vi "oa_If Param Changed, Set Reset True (1 Channel).vi"(0 "scaled signal in [EU]":waveform(dbl)={"t0"=timestamp(0 s since 1904-01-01), "dt"=0.0, "Y"=[]}, 1 "reset in":bool=TRUE, 5 "speed profile":T1 {"speed [RPM]" format="%.2f"; "time [s]" format="%.2f"}, 7 "pulse/revolution in (1)":i32=1, 9 "max order in (auto)":dbl, 11 "error in (no error)":errorcluster, 12 "analysis method in":u16(ring) items=["fast", "accurate"]) -> (3 "reset out":bool=TRUE, 4 "scaled signal out [EU]":waveform(dbl), 6 "speed profile out":T1 {"speed [RPM]" format="%.2f"; "time [s]" format="%.2f"}, 8 "pulse/revolution out (1)":i32=1, 10 "max order out (auto)":dbl, 14 "analysis method out":u16(ring) items=["fast", "accurate"], 15 "error out":errorcluster)   [LabVIEW 2017, in "SoundVib_Resampling.lvlib"]
uses:
  <vilib>/addons/Sound and Vibration/Order Analysis/Resample Order Tracking/SoundVib_Resampling.lvlib
  <vilib>/addons/Sound and Vibration/Order Analysis/Tach Process/SubVIs/speed profile.ctl
  <vilib>/addons/Sound and Vibration/Order Analysis/Tach Process/SoundVib_TachProcess.lvlib
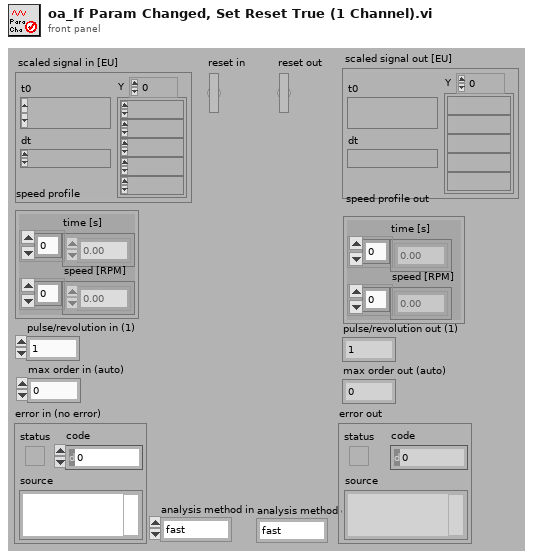
[diagram p1: front panel]
types:
  T1 = typedef "SoundVib_TachProcess.lvlib/speed profile.ctl" = cluster{"time [s]":dbl[], "speed [RPM]":dbl[]}
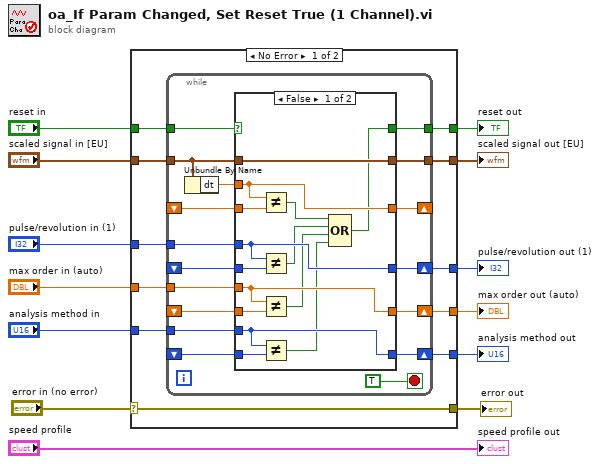
[diagram p0: block diagram]
diagram:
  n1 = case shown="No Error" "error in (no error)" {
    selector: "error in (no error)" -> [w14 w67]
    tunnel: "max order in (auto)" -> [w24 w63]
    tunnel: "reset in" -> [w23 w66]
    tunnel: [w22 w66] -> w11
    tunnel: [w21 w65] -> w10
    tunnel: "pulse/revolution in (1)" -> [w20 w64]
    tunnel: [w19 w64] -> w8
    tunnel: [w18 w63] -> w7
    tunnel: "analysis method in" -> [w17 w62]
    tunnel: [w16 w62] -> w5
    tunnel: "scaled signal in [EU]" -> [w15 w65]
    tunnel: [w14 w67] -> w1
    frame No Error {
      n2 = while {
        tunnel: w24 -> [w41]
        tunnel: w23 -> [w40]
        tunnel: [w39] -> w22
        tunnel: w15 -> [w31]
        tunnel: [w38] -> w21
        tunnel: w20 -> [w37]
        tunnel: w17 -> [w34]
        shift-right: [w36] -> w19
        shift-left: _ -> [w27]
        shift-right: [w35] -> w18
        shift-left: _ -> [w26]
        shift-right: [w33] -> w16
        shift-left: _ -> [w25]
        shift-right: [w29] -> _
        shift-left: _ -> [w28]
        stop <- TRUE stop-if-true
        n3 = Unbundle By Name(w31) -> ("dt"=w30:dbl)
        n4 = case shown="False" w40 {
          selector: w40 -> [_ w61]
          tunnel: w41 -> [w50 w58]
          tunnel: [w42 w61] -> w39
          tunnel: w31 -> [w55 w60]
          tunnel: [w55 w60] -> w38
          tunnel: w37 -> [w52 w59]
          tunnel: [w52 w59] -> w36
          tunnel: [w50 w58] -> w35
          tunnel: w34 -> [w47 w57]
          tunnel: [w47 w57] -> w33
          tunnel: w30 -> [w54 w56]
          tunnel: [w54 w56] -> w29
          tunnel: w28 -> [w53 _]
          tunnel: w27 -> [w51 _]
          tunnel: w26 -> [w49 _]
          tunnel: w25 -> [w48 _]
          frame False {
            n5 = Not Equal?(x=w54, y=w53) -> (x != y?=w46:bool)
            n6 = Not Equal?(x=w52, y=w51) -> (x != y?=w45:bool)
            n7 = Not Equal?(x=w50, y=w49) -> (x != y?=w44:bool)
            n8 = Not Equal?(x=w47, y=w48) -> (x != y?=w43:bool)
            n9 = Compound Arithmetic op=OR(w46, w45, w44, w43) -> (w42:bool)
          }
          frame True {
          }
        }
      }
    }
    frame Error {
    }
  }
  "reset out" <- w11
  "scaled signal out [EU]" <- w10
  "pulse/revolution out (1)" <- w8
  "analysis method out" <- w5
  "max order out (auto)" <- w7
  "error out" <- w1
  "speed profile out" <- "speed profile"
